vi "RampVoltagewithDDSv4.vi"() -> ()   [LabVIEW 2016]
uses:
  <vilib>/DAQmx/write.llb/DAQmx Write (Analog 2D DBL NChan NSamp).vi
  <vilib>/DAQmx/create/channels.llb/DAQmx Create Channel (AO-Voltage-Basic).vi
  <vilib>/DAQmx/configure/timing.llb/DAQmx Timing (Sample Clock).vi
  <vilib>/DAQmx/configure/trigger.llb/DAQmx Start Trigger (Digital Edge).vi
  <vilib>/DAQmx/miscellaneous.llb/DAQmx Fill In Error Info.vi
  <resource>/objmgr/daqmx.rc
panel:
  in  "physical channels 3":tag="Dev4/ao2"
  out "appended array":dbl[](array[numeric])
  in  "Sinewave amp (V)":dbl=2.0 format="%#_6f"
  in  "Sinewave duration (ms)":dbl=0.3 format="%#_13g"
  out "size(s)":i32=7026
  in  "Trigger delay NI (ms)":dbl
  out "Sample rate":dbl=502512.5628140703
  in  "Trigger delay DDS (ms)":dbl=0.22 step=0.01 format="%#_13g"
  in  "source":tag="/Dev4/PFI0"
  in  "physical channels 2":tag="Dev4/ao1"
  in  "physical channels":tag="Dev4/ao0"
  in  "Plateau time (ms)":dbl=10.0
  out "Step seperation (us)":dbl=0.40857142857142853
  in  "Ramp duration (us)":dbl=2002.0 format="%#_6f"
  in  "Ramp trigger source":T1(ring)=enum."BNC_IN_A_RISING"
  in  "Step Size (Hz)":dbl=10000.0 format="%#_6f"
  in  "End Frequency (Hz)":dbl=250000000.0 format="%#_13g"
  in  "Starting Frequency (Hz)":dbl=201000000.0 format="%#_6f"
  in  "Channels":T2(ring)=enum."Both channels"
  out "return count":u32=352
  out "error out":errorcluster={"status"=TRUE, "code"=-1073807339, "source"="VISA Read in RampVoltagewithDDSv3.vi"}
  out "read buffer":string="dcp spi:CFR2=0x1000080\r\nflexdds> dcp spi:STP0=0x3FFF00003374BC6A\r\nflexdds> dcp wait::BNC_IN_A_RISING\r\nflexdds> dcp update:u\r\nflexdds> dcp spi:DRL=0x400000003374BC6A\r\nflexdds> dcp spi:DRSS=0xA7C60000A7C6\r\nflexdds> dcp spi:DRR=0x660066\r\nflexdds> dcp spi:CFR2=0x80080\r\nflexdds> dcp wait:0h:\r\nflexdds> dcp update:u+d\r\nflexdds> dcp wait:1500250h:\r\nflexdds> dcp update:-d\r\nflexdds> dcp spi:CFR2=0x1000080\r\nflexdds> dcp spi:STP0=0x3FFF00003374BC6A\r\nflexdds> dcp wait:250250h:\r\nflexdds> dcp update:u\r\nflexdds> dcp start\r\n\u001b[34m[ 250351127 N shell] L:FPGA:DCP[0]: flushing 20 insts (120 bytes); FIFO 0/4096 ent..."
  out "Final instruction string":string="dcp spi:CFR2=0x1000080\rdcp spi:STP0=0x3FFF00003374BC6A\rdcp wait::BNC_IN_A_RISING\rdcp update:u\rdcp spi:DRL=0x400000003374BC6A\rdcp spi:DRSS=0xA7C60000A7C6\rdcp spi:DRR=0x660066\rdcp spi:CFR2=0x80080\rdcp wait:0h:\rdcp update:u+d\rdcp wait:1500250h:\rdcp update:-d\rdcp spi:CFR2=0x1000080\rdcp spi:STP0=0x3FFF00003374BC6A\rdcp wait:250250h:\rdcp update:u\rdcp start\r"
  in  "Plateau duration (ms)":dbl=10.0
  in  "Ramp duration (ms)":dbl=1.99 step=0.01
  in  "No of samples in ramp":dbl=1000.0
  in  "Ramp Amplitude (V)}":dbl=0.044 step=0.001
  in  "error in":errorcluster
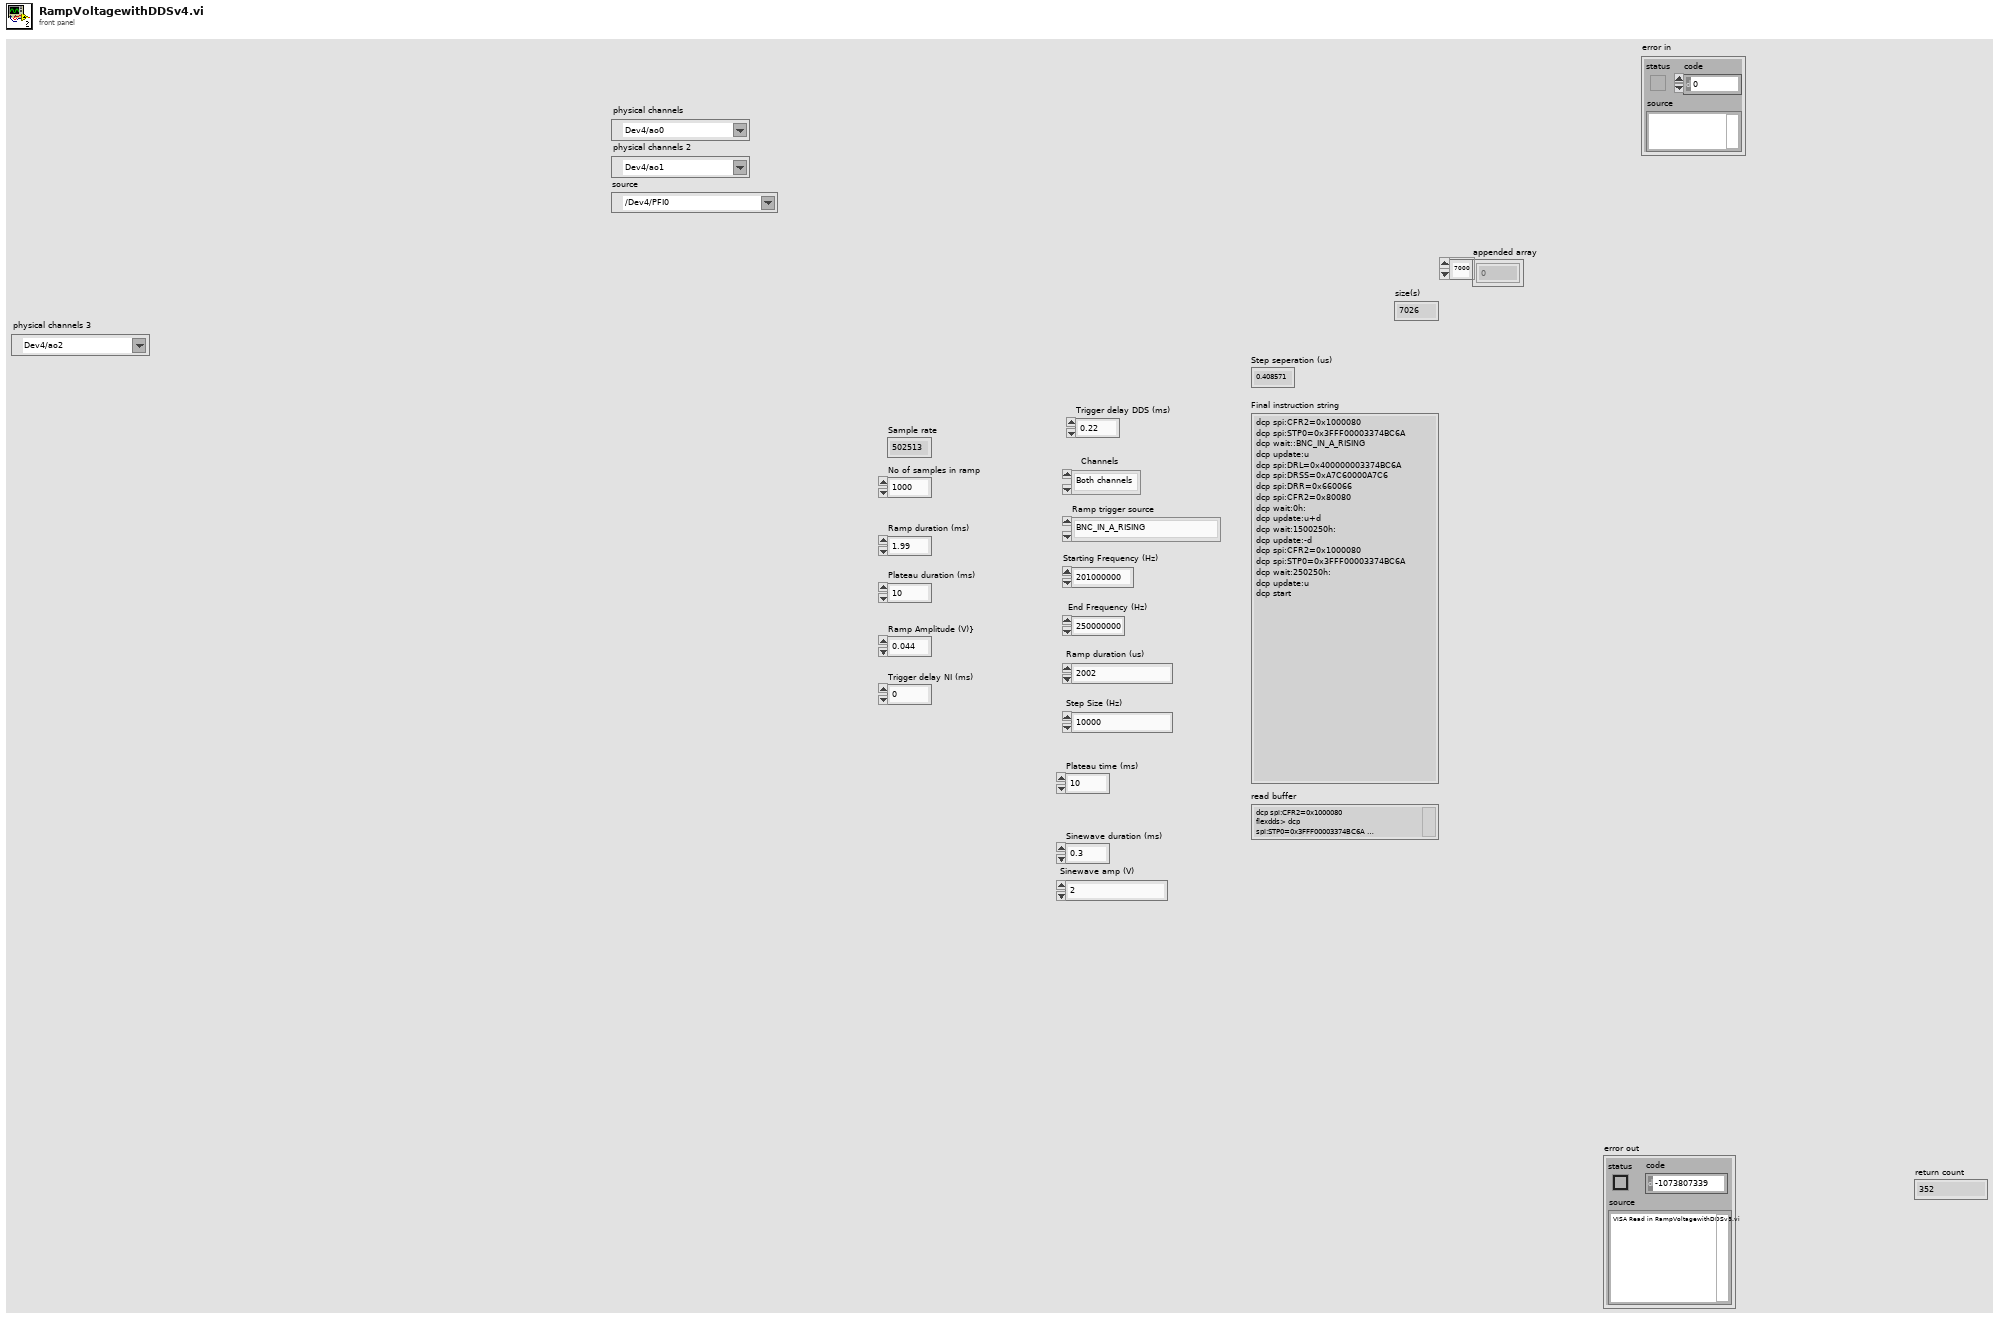
[diagram p1: front panel]
types:
  T1 = enum32{"O_RAMP_SWP_OVR", "RAM_SWP_OVR", "O_DROVER", "DROVER", "O_SPI_FIFO_EV1", "SPI_FIFO_EV1", "O_SPI_FIFO_EV0", "SPI_FIFO_EV0", "O_SPI_FIFO_FLUSHED", "SPI_FIFO_FLUSHED", "BNC_IN_B_LEVEL", "BNC_IN_B_FALLING", "BNC_IN_B_RISING", "BNC_IN_A_LEVEL", "BNC_IN_A_FALLING", "BNC_IN_A_RISING", "ALL_SPI_FIFOS_FLUSHED", "NONE"}
  T2 = enum32{"Channel 0", "Channel 1", "Both channels"}
  T3 = cluster{"Enable ASF from STP (F)":bool, "Digital ramp enable (F)":bool, "Digital ramp no-dwell high (F)":bool, "Digital ramp no-dwell low (F)":bool, "Matched latency enable (T)":bool, "Parallel data port enable (F)":bool}
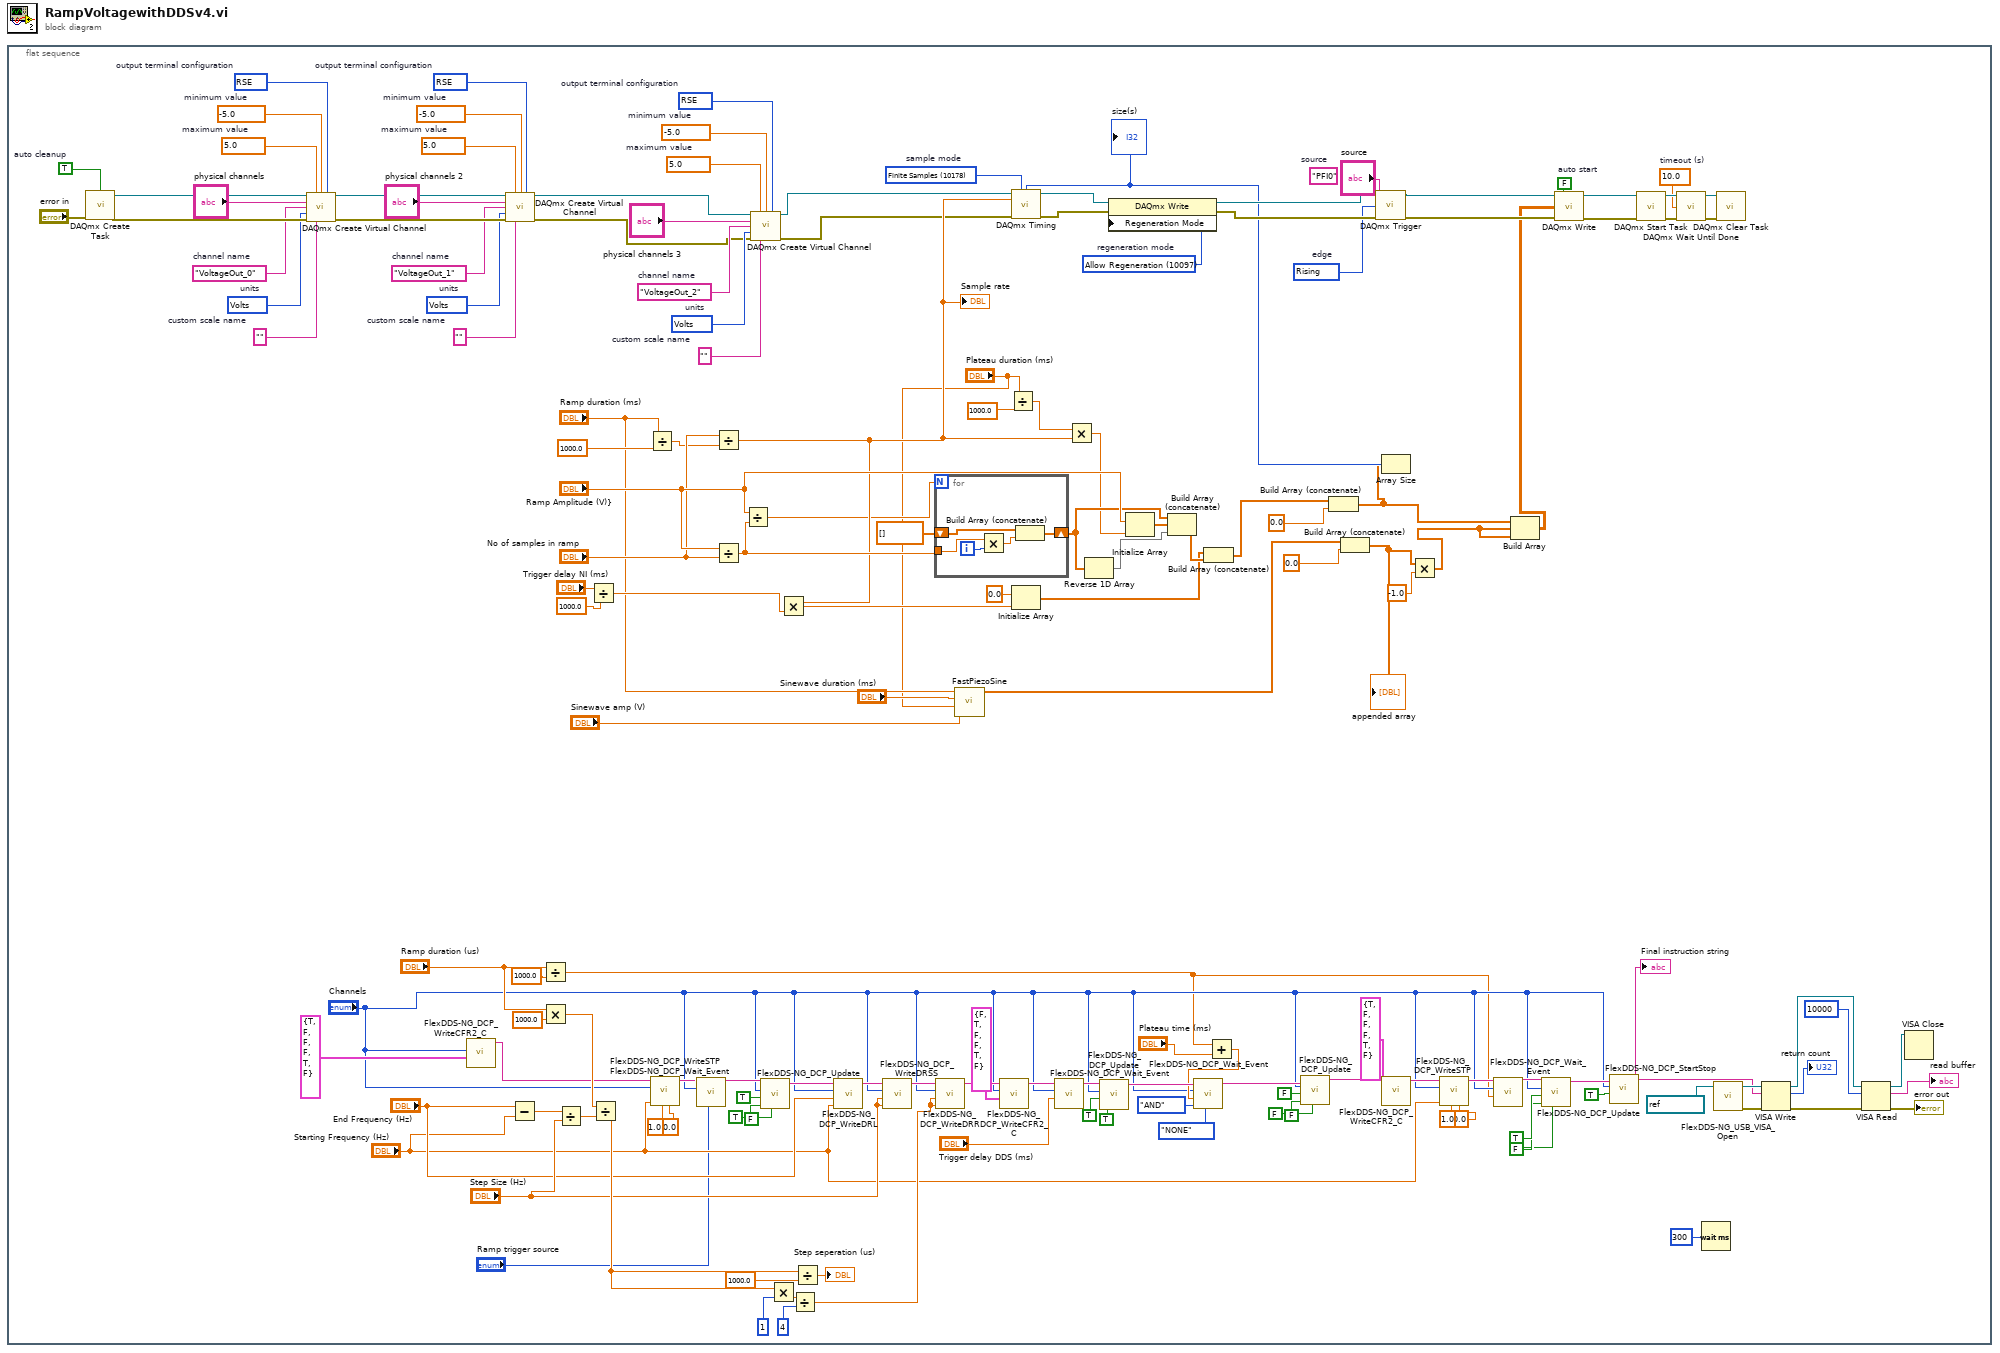
[diagram p0: block diagram]
diagram:
  n1 = flat-sequence {
    frame #0 {
      w9 = 10083 items=["Default"=-1, "RSE"=10083, "Differential"=10106, "Pseudodifferential"=12529]  # output terminal configuration
      w10 = 10348 items=["Volts"=10348, "From Custom Scale"=10065]  # units
      w11 = "VoltageOut_2"  # channel name
      w12 = ""  # custom scale name
      w13 = -5.0  # minimum value
      w14 = 5.0  # maximum value
      w123 = 10280 items=["Rising"=10280, "Falling"=10171]  # edge
      (unwired) "PFI0"  # source
      w125 = 10097 items=["Allow Regeneration"=10097, "Do Not Allow Regeneration"=10158]  # regeneration mode
      w128 = 10178 items=["Finite Samples"=10178, "Continuous Samples"=10123, "Hardware Timed Single Point"=12522]  # sample mode
      w130 = 10083 items=["Default"=-1, "RSE"=10083, "Differential"=10106, "Pseudodifferential"=12529]  # output terminal configuration
      w131 = 10348 items=["Volts"=10348, "From Custom Scale"=10065]  # units
      w132 = "VoltageOut_1"  # channel name
      w133 = ""  # custom scale name
      w134 = -5.0  # minimum value
      w135 = 5.0  # maximum value
      w137 = 10083 items=["Default"=-1, "RSE"=10083, "Differential"=10106, "Pseudodifferential"=12529]  # output terminal configuration
      w138 = 10348 items=["Volts"=10348, "From Custom Scale"=10065]  # units
      w139 = "VoltageOut_0"  # channel name
      w141 = ""  # custom scale name
      w142 = -5.0  # minimum value
      w143 = 5.0  # maximum value
      w145 = TRUE  # auto cleanup
      w151 = 10.0  # timeout (s)
      w155 = FALSE  # auto start
      n2 = call <vilib>:"DAQmx Create Task.vi"("auto cleanup"=w145, "error in"="error in") -> ("task out"=w144:refnum<k21>, "error out"=w146:errorcluster)  [unwired: 12 in]
      n3 = call-poly <vilib>:"DAQmx Create Virtual Channel.vi"("task in"=w144, "maximum value"=w143, "minimum value"=w142, "output terminal configuration"=w137, "physical channels"="physical channels", "name to assign"=w139, "units"=w138, "error in"=w146, "custom scale name"=w141) -> ("task out"=w136:refnum<k21>, "error out"=w140:errorcluster)  [unwired: 5 in]
      n4 = call "FlexDDS-NG_DCP_WriteCFR2_C.vi"("CFR2 bits"=T3 {"Enable ASF from STP (F)"=TRUE, "Digital ramp enable (F)"=FALSE, "Digital ramp no-dwell high (F)"=FALSE, "Digital ramp no-dwell low (F)"=FALSE, "Matched latency enable (T)"=TRUE, "Parallel data port enable (F)"=FALSE} ("CFR2 bits 2"), "Channels"="Channels") -> ("appended instruction string"=w57:string)  [unwired: 9 in]
      n5 = call-poly <vilib>:"DAQmx Create Virtual Channel.vi"("task in"=w136, "maximum value"=w135, "minimum value"=w134, "output terminal configuration"=w130, "physical channels"="physical channels 2", "name to assign"=w132, "units"=w131, "error in"=w140, "custom scale name"=w133) -> ("task out"=w7:refnum<k21>, "error out"=w6:errorcluster)  [unwired: 5 in]
      n6 = Subtract(x="End Frequency (Hz)", y="Starting Frequency (Hz)") -> (x-y=w69:dbl)
      n7 = Divide(x="Ramp duration (us)", y=1000.0) -> (x/y=w38:dbl)
      n8 = Multiply(x="Ramp duration (us)", y=1000.0) -> (x*y=w66:dbl)
      n9 = Divide(x=w69, y="Step Size (Hz)") -> (x/y=w67:dbl)
      n10 = Divide(x="Trigger delay NI (ms)", y=1000.0) -> (x/y=w29:dbl)
      n11 = Divide(x=w66, y=w67) -> (x/y=w65:dbl)
      n12 = Divide(x="Ramp duration (ms)", y=1000.0) -> (x/y=w114:dbl)
      n13 = call "FlexDDS-NG_DCP_WriteSTP.vi"("phase degrees (0..360)"=0.0, "amplitude (0..1)"=1.0, "frequency Hz (0..400M)"="Starting Frequency (Hz)", "Channels"="Channels", "initial instruction string"=w57) -> ("appended instruction string"=w52:string)  [unwired: 6 in]
      n14 = call "FlexDDS-NG_DCP_Wait_Event.vi"("Event 1"="Ramp trigger source", "Channels in"="Channels", "appended instruction string in"=w52) -> ("appended instruction string"=w53:string)  [unwired: 8 in]
      n15 = Divide(x="No of samples in ramp", y=w114) -> (x/y=w28:dbl)
      "Sample rate" <- w28
      n16 = Divide(x="Ramp Amplitude (V)}", y="No of samples in ramp") -> (x/y=w121:dbl)
      n17 = Divide(x="Ramp Amplitude (V)}", y=w121) -> (x/y=w25:dbl)
      n18 = call-poly <vilib>:"DAQmx Create Virtual Channel.vi"("task in"=w7, "maximum value"=w14, "minimum value"=w13, "output terminal configuration"=w9, "physical channels"="physical channels 3", "name to assign"=w11, "units"=w10, "error in"=w6, "custom scale name"=w12) -> ("task out"=w5:refnum<k21>, "error out"=w4:errorcluster)  [unwired: 5 in]
      n19 = call "FlexDDS-NG_DCP_Update.vi"("ONLY IO_UPDATE"=TRUE, "DRCTL(true=+, false=-)"=FALSE ("DRCTL(true=+, false=-) 2"), "IO_UPDATE(true=u, false = '')"=TRUE ("IO_UPDATE(true=u, false = '')  2"), "Channels"="Channels", "appended instruction string in"=w53) -> ("appended instruction string out"=w51:string)  [unwired: 6 in]
      n20 = Multiply(x=w65, y=u16 1) -> (x*y=w71:dbl)
      n21 = Multiply(x=w28, y=w29) -> (x*y=w27:dbl)
      n22 = Divide(x=w71, y=u16 4) -> (x/y=w45:dbl)
      n23 = Divide(x=w65, y=1000.0 ("x/y")) -> (x/y=→"Step seperation (us)":dbl)
      n24 = call "FlexDDS-NG_DCP_WriteDRL.vi"("low limit"="Starting Frequency (Hz)", "high limit"="End Frequency (Hz)", "Channels"="Channels", "initial instruction string"=w51) -> ("appended instruction string"=w94:string)  [unwired: 7 in]
      n25 = call "FlexDDS-NG_DCP_WriteDRSS.vi"("increment step size"="Step Size (Hz)", "decrement step size"="Step Size (Hz)", "Channels"="Channels", "initial instruction string"=w94) -> ("appended instruction string"=w93:string)  [unwired: 7 in]
      n26 = for {
        N: w25 -> [_]
        shift-right: [w158] -> w119
        shift-left: dbl[] [] -> [w157]
        tunnel: w121 -> [w156]
        i -> [w160]
        n27 = Multiply(x=w156, y=w160) -> (x*y=w159:dbl)
        n28 = Build Array (concatenate)(w157, w159) -> (w158:dbl[])
      }
      n29 = call "FlexDDS-NG_DCP_WriteDRR.vi"("digital ramp positive slope rate"=w45, "digital ramp negative slope rate"=w45, "Channels"="Channels", "initial instruction string"=w93) -> ("appended instruction string"=w92:string)  [unwired: 7 in]
      n30 = call "FastPiezoSine.vi"("Sinewave amp (V)"="Sinewave amp (V)", "Plateau duration (ms)"="Plateau duration (ms)", "Sinewave duration (ms)"="Sinewave duration (ms)", "Ramp duration (ms)"="Ramp duration (ms)") -> ("appended array"=w18:dbl[])  [unwired: 7 in]
      n31 = call "FlexDDS-NG_DCP_WriteCFR2_C.vi"("CFR2 bits"=T3 {"Enable ASF from STP (F)"=FALSE, "Digital ramp enable (F)"=TRUE, "Digital ramp no-dwell high (F)"=FALSE, "Digital ramp no-dwell low (F)"=FALSE, "Matched latency enable (T)"=TRUE, "Parallel data port enable (F)"=FALSE}, "Channels"="Channels", "initial instruction string"=w92) -> ("appended instruction string"=w87:string)  [unwired: 8 in]
      n32 = Divide(x="Plateau duration (ms)", y=1000.0) -> (x/y=w110:dbl)
      n33 = Initialize Array(0.0 ("element"), w27) -> (w34:dbl[])
      n34 = call "FlexDDS-NG_DCP_Wait_Event.vi"("waiting time [ms]"="Trigger delay DDS (ms)", "Channels in"="Channels", "appended instruction string in"=w87) -> ("appended instruction string"=w86:string)  [unwired: 8 in]
      n35 = Multiply(x=w110, y=w28) -> (x*y=w109:dbl)
      n36 = Reverse 1D Array(array=w119) -> (reversed array=w117:dbl[])
      n37 = call "FlexDDS-NG_DCP_Update.vi"("DRCTL(true=+, false=-)"=TRUE, "IO_UPDATE(true=u, false = '')"=TRUE, "Channels"="Channels", "appended instruction string in"=w86) -> ("appended instruction string out"=w82:string)  [unwired: 7 in]
      n38 = Initialize Array("Ramp Amplitude (V)}", w109) -> (w118:dbl[])
      n39 = Build Array (concatenate)(w119, w118, w117) -> (w35:dbl[])
      n40 = Build Array (concatenate)(w34, w35) -> (w21:dbl[])
      n41 = Add(x=w38, y="Plateau time (ms)") -> (x+y=w42:dbl)
      n42 = call "FlexDDS-NG_DCP_Wait_Event.vi"("Event 1"=T1."NONE", "AND/OR"=enum32{"AND", "OR"}."AND", "waiting time [ms]"=w42, "Channels in"="Channels", "appended instruction string in"=w82) -> ("appended instruction string"=w41:string)  [unwired: 6 in]
      n43 = call "FlexDDS-NG_DCP_Update.vi"("ONLY IO_UPDATE"=FALSE, "DRCTL(true=+, false=-)"=FALSE ("DRCTL(true=+, false=-) 2"), "IO_UPDATE(true=u, false = '')"=FALSE ("IO_UPDATE(true=u, false = '')  2"), "Channels"="Channels", "appended instruction string in"=w41) -> ("appended instruction string out"=w43:string)  [unwired: 6 in]
      n44 = Build Array (concatenate)(w21, 0.0 ("y")) -> (w17:dbl[])
      n45 = Build Array (concatenate)(w18, 0.0 ("y")) -> (w16:dbl[])
      "appended array" <- w16
      n46 = Array Size(array=w17) -> (size(s)=w108:i32)
      "size(s)" <- w108
      n47 = call-poly <vilib>:"DAQmx Timing.vi"("task/channels in"=w5, "sample mode"=w128, "samples per channel"=w108, "rate"=w28, "error in"=w4) -> ("task out"=w127:refnum<k21>, "error out"=w129:errorcluster)  [unwired: 9 in]
      n48 = property class="DAQmx Write"(reference=w127, error in=w129, "Regeneration Mode"=w125) -> (reference out=w124:refnum<k21>, error out=w126:errorcluster)
      n49 = call-poly <vilib>:"DAQmx Trigger.vi"("task/channels in"=w124, "source"="source", "edge"=w123, "error in"=w126) -> ("task out"=w113:refnum<k21>, "error out"=w112:errorcluster)  [unwired: 10 in]
      n50 = call "FlexDDS-NG_DCP_WriteCFR2_C.vi"("CFR2 bits"=T3 {"Enable ASF from STP (F)"=TRUE, "Digital ramp enable (F)"=FALSE, "Digital ramp no-dwell high (F)"=FALSE, "Digital ramp no-dwell low (F)"=FALSE, "Matched latency enable (T)"=TRUE, "Parallel data port enable (F)"=FALSE}, "initial instruction string"=w43) -> ("appended instruction string"=w75:string)  [unwired: 9 in]
      n51 = Multiply(x=w16, y=-1.0 ("element")) -> (x*y=w3:dbl[])
      n52 = call "FlexDDS-NG_DCP_WriteSTP.vi"("phase degrees (0..360)"=0.0, "amplitude (0..1)"=1.0, "frequency Hz (0..400M)"="Starting Frequency (Hz)", "Channels"="Channels", "initial instruction string"=w75) -> ("appended instruction string"=w74:string)  [unwired: 6 in]
      n53 = call "FlexDDS-NG_DCP_Wait_Event.vi"("waiting time [ms]"=w38, "Channels in"="Channels", "appended instruction string in"=w74) -> ("appended instruction string"=w73:string)  [unwired: 8 in]
      n54 = Build Array(w17, w3, w3) -> (w26:dbl[][])
      n55 = call "FlexDDS-NG_DCP_Update.vi"("ONLY IO_UPDATE"=TRUE, "DRCTL(true=+, false=-)"=FALSE ("DRCTL(true=+, false=-) 2"), "IO_UPDATE(true=u, false = '')"=TRUE ("IO_UPDATE(true=u, false = '')  2"), "Channels"="Channels", "appended instruction string in"=w73) -> ("appended instruction string out"=w78:string)  [unwired: 6 in]
      n56 = call-poly <vilib>:"DAQmx Write.vi"("task/channels in"=w113, "auto start"=w155, "data"=w26, "error in"=w112) -> ("task out"=w150:refnum<k21>, "error out"=w149:errorcluster)  [unwired: 9 in, 1 out]
      n57 = call "FlexDDS-NG_DCP_StartStop.vi"("start (T) stop (F)"=TRUE, "Channels"="Channels", "initial instruction string"=w78) -> ("appended instruction string"=w50:string)  [unwired: 8 in]
      "Final instruction string" <- w50
      n58 = call <vilib>:"DAQmx Start Task.vi"("task/channels in"=w150, "error in"=w149) -> ("task out"=w154:refnum<k21>, "error out"=w153:errorcluster)  [unwired: 12 in]
      n59 = call <vilib>:"DAQmx Wait Until Done.vi"("task/channels in"=w154, "timeout (sec)"=w151, "error in"=w153) -> ("task out"=w148:refnum<k21>, "error out"=w152:errorcluster)  [unwired: 11 in]
      n60 = Wait (ms)(milliseconds to wait=u32 300) -> ()  [unwired: 1 out]
      n61 = call "FlexDDS-NG_USB_VISA_Open.vi"("FlexDDS-NG USB VISA resource name (COM)"=refnum<visa-resource-name> "COM7") -> ("error out"=w96:errorcluster, "FlexDDS-NG USB VISA resource name out"=w97:refnum<visa-resource-name>)  [unwired: 9 in]
      n62 = call <vilib>:"DAQmx Clear Task.vi"("task in"=w148, "error in"=w152) -> ()  [unwired: 13 in, 1 out]
      n63 = VISA Write(VISA resource name=w97, write buffer=w50, error in (no error)=w96) -> (VISA resource name out=w101:refnum<visa-resource-name>, return count=→"return count":u32, error out=w99:errorcluster)
      n64 = VISA Read(VISA resource name=w101, byte count=u32 10000, error in (no error)=w99) -> (VISA resource name out=w104:refnum<visa-resource-name>, read buffer=→"read buffer":string, error out=→"error out":errorcluster)  [unwired: 1 out]
      n65 = VISA Close(VISA resource name=w104) -> ()  [unwired: 1 in, 1 out]
    }
  }
